vi "Adressen.vi"(8 "error in (no error)":errorcluster caption="Fehler (Eingang, kein Fehler)", 11 "mini8 Steuerung PNS Eingang":refnum<class "mini8 Steuerung PNS.lvclass">) -> (0 "error out":errorcluster caption="Fehler (Ausgang)", 2 "Adressen out":T1, 3 "mini8 Steuerung PNS Ausgang":refnum<class "mini8 Steuerung PNS.lvclass">)   [LabVIEW 2020, in "mini8 Steuerung PNS.lvclass"]
uses:
  mini8 Steuerung PNS.lvclass
  Adresse.ctl
  Steuerung PNS.lvclass
panel:
  out "Alarm":u16[](array[numeric])
  out "Allgemein":u16[](array[numeric])
  out "Heizkreiserkennung":u16[](array[numeric])
  out "Loop1":u16[](array[numeric])
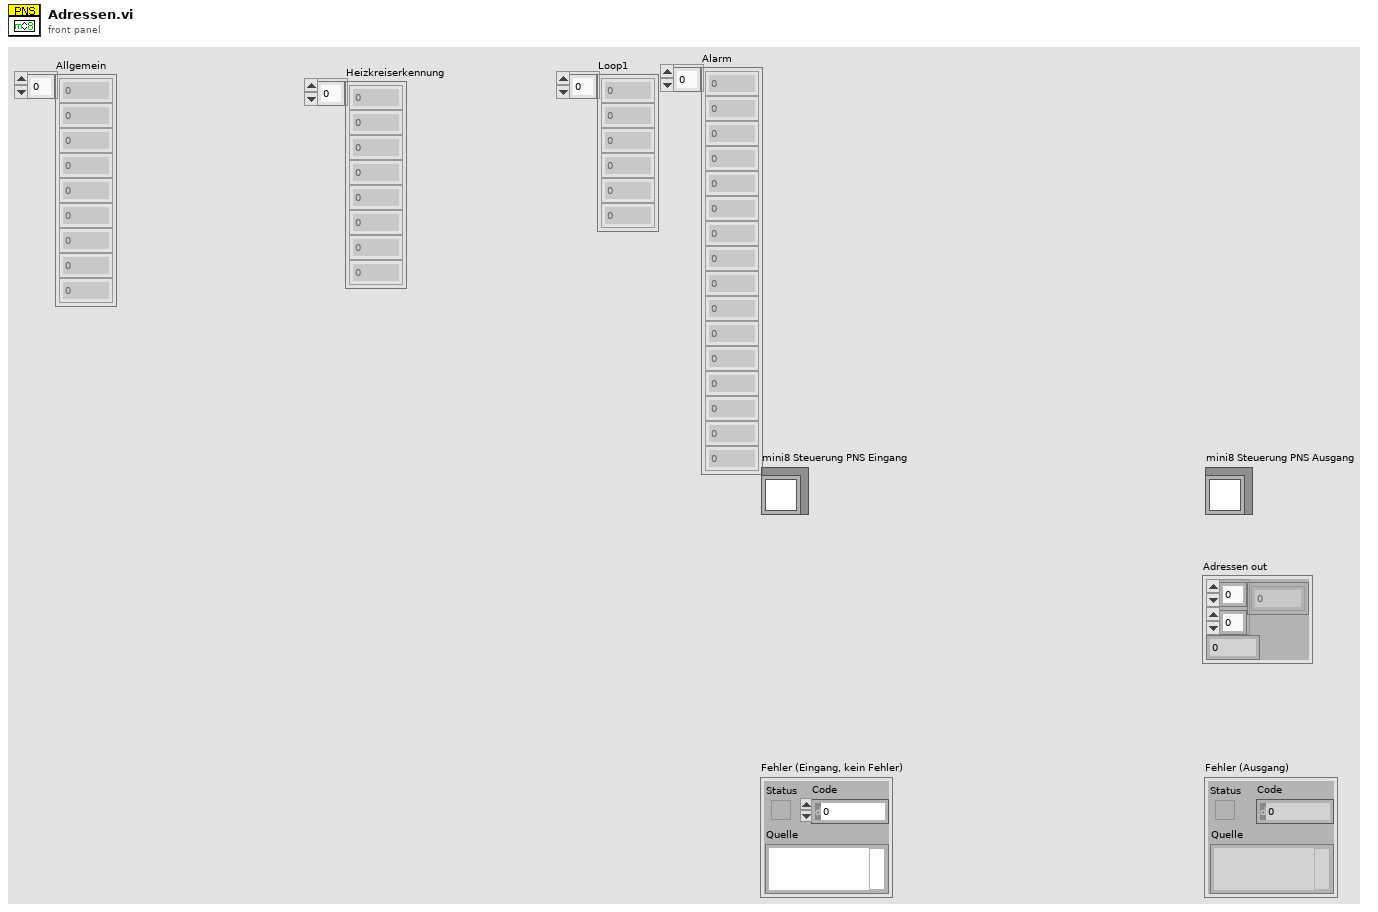
[diagram p1: front panel]
types:
  T1 = typedef "Steuerung PNS.lvclass/Adresse.ctl" = cluster{i32[][], i32}
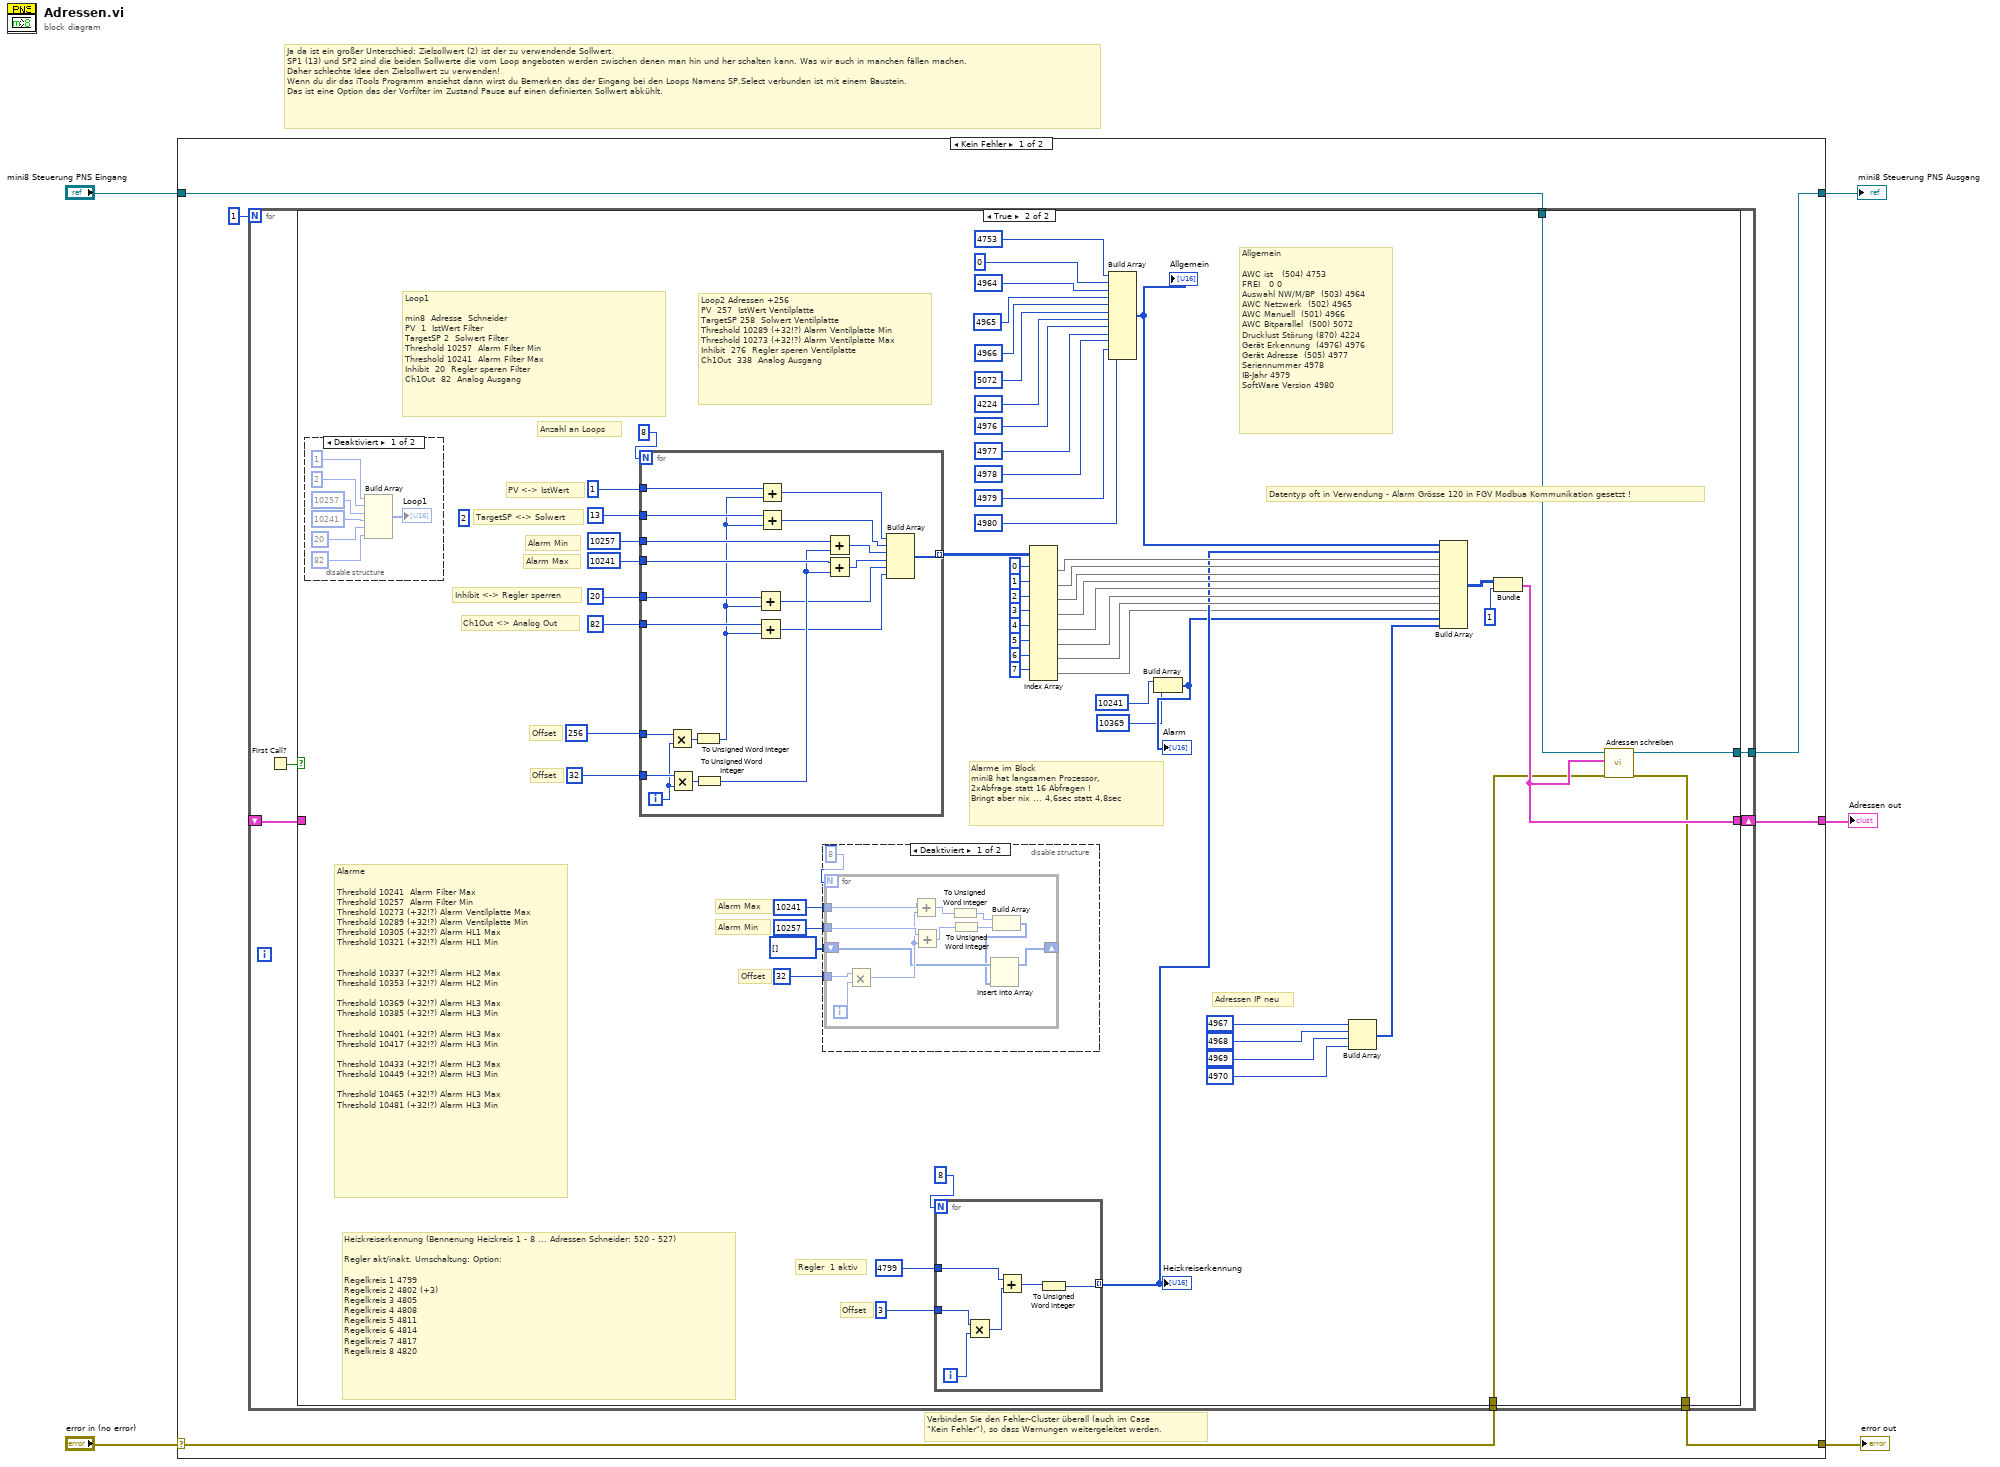
[diagram p0: block diagram]
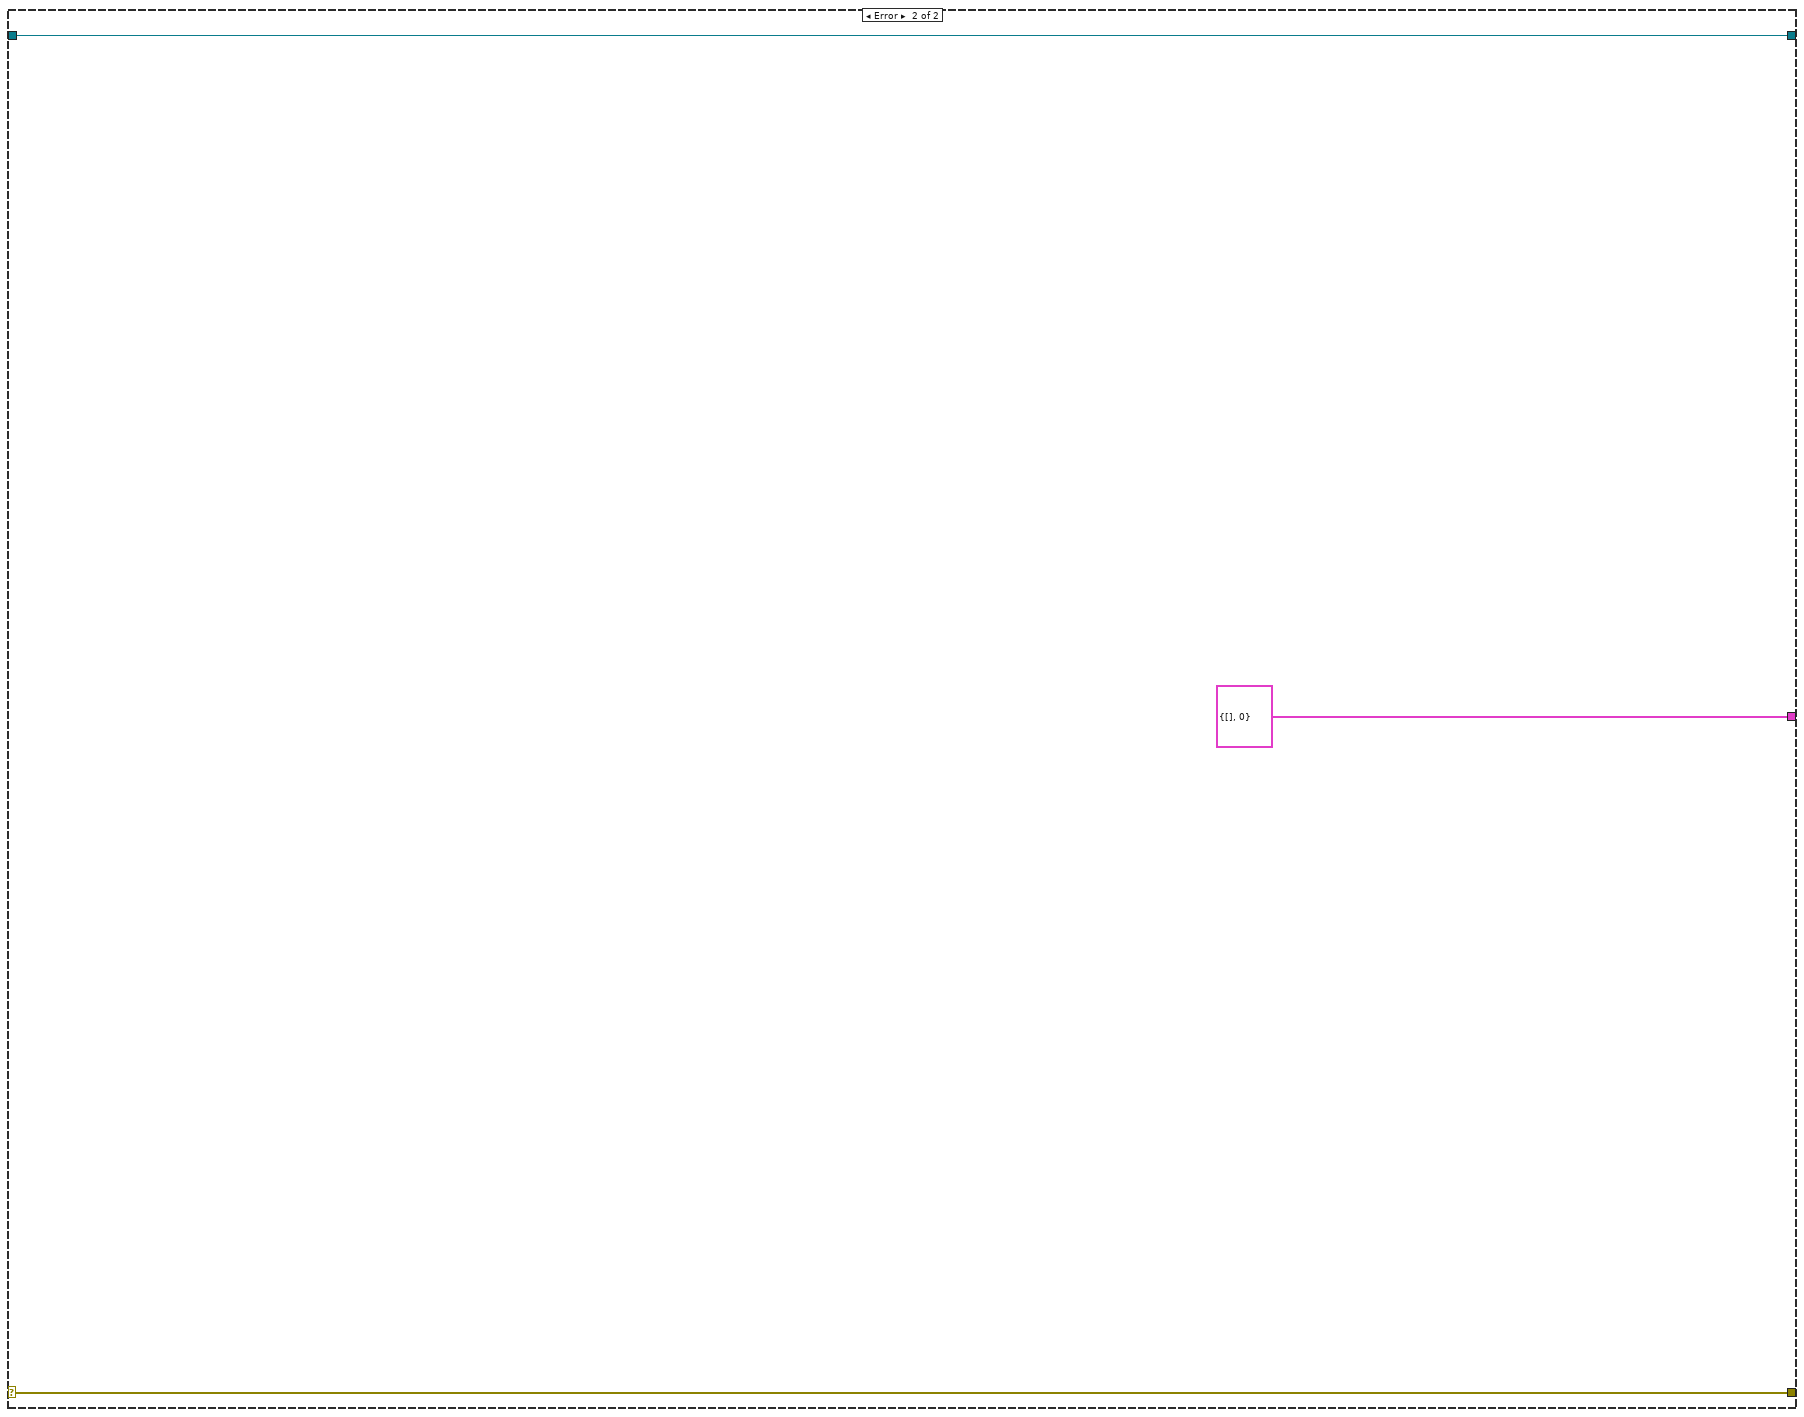
[diagram p5: hidden frame]
diagram:
  # "Ja da ist ein großer Unterschied: Zielsollwert (2) ist der zu verwendende Sollwert.\nSP1 (13) und SP2 sind die beiden Sollwerte die vom Loop angeboten werden zwischen denen man hin und her schalten kann. Was wir auch in manchen fällen machen. \nDaher schlechte Idee den Zielsollwert zu verwenden!\nWenn du dir das iTools Programm ansiehst dann wirst du Bemerken das der Eingang bei den Loops Namens SP.Select verbunden ist mit einem Baustein.\nDas ist eine Option das der Vorfilter im Zustand Pause auf einen definierten Sollwert abkühlt."
  n1 = case shown="Kein Fehler" "error in (no error)" {
    selector: "error in (no error)" -> [w7 w136]
    tunnel: [w6 w136] -> w4
    tunnel: [w8 w135] -> w2
    tunnel: "mini8 Steuerung PNS Eingang" -> [w9 w135]
    tunnel: [w11 cluster{i32[][], i32} {[], 0} ("Adressen out")] -> w1
    frame No Error {
      # "Verbinden Sie den Fehler-Cluster überall (auch im Case\n\"Kein Fehler\"), so dass Warnungen weitergeleitet werden."
      n2 = for {
        N: 1 -> [_]
        shift-right: [w17] -> w11
        shift-left: _ -> [w16]
        tunnel: [w14] -> w8
        tunnel: w9 -> [w15]
        tunnel: w7 -> [w13]
        tunnel: [w12] -> w6
        n3 = First Call?() -> (First Call?: T/F=w18:bool)
        n4 = case shown="True" w18 {
          tunnel: [w21 w35] -> w17
          tunnel: w16 -> [w21 _]
          tunnel: w15 -> [w20 w33]
          tunnel: [w20 w34] -> w14
          tunnel: w13 -> [w19 w32]
          tunnel: [w19 w31] -> w12
          frame False {
          }
          frame True {
            (unwired) u16 2 ("Numerisches Element")
            # "Adressen IP neu"
            # "Datentyp oft in Verwendung - Alarm Grösse 120 in FGV Modbua Kommunikation gesetzt !"
            # "Alarme im Block\nmini8 hat langsamen Prozessor,\n2xAbfrage statt 16 Abfragen !\nBringt aber nix ... 4,6sec statt 4,8sec"
            # "Allgemein\n\nAWC ist\t\t\t(504)\t4753\nFREI\t\t\t0\t0\nAuswahl NW/M/BP\t\t(503)\t4964\nAWC Netzwerk\t\t(502)\t4965\nAWC Manuell\t\t(501)\t4966\nAWC Bitparallel\t\t(500)\t5072\nDrucklust Störung\t(870)\t4224\nGerät Erkennung\t\t(4976)\t4976\nGerät Adresse\t\t(505)\t4977\nSeriennummer 4978\nIB-Jahr 4979\nSoftWare Version 4980"
            # "Offset"
            # "Regler  1 aktiv"
            # "Heizkreiserkennung (Bennenung Heizkreis 1 - 8 ... Adressen Schneider: 520 - 527)\n\nRegler akt/inakt. Umschaltung: Option:\n\nRegelkreis 1\t4799\nRegelkreis 2\t4802 (+3)\nRegelkreis 3\t4805\nRegelkreis 4\t4808\nRegelkreis 5\t4811\nRegelkreis 6\t4814\nRegelkreis 7\t4817\nRegelkreis 8\t4820"
            # "Alarm Min"
            # "Alarm Max"
            # "Offset"
            # "Alarme\n\nThreshold\t10241\t\tAlarm Filter Max\nThreshold\t10257\t\tAlarm Filter Min\nThreshold\t10273\t(+32!?)\tAlarm Ventilplatte Max\nThreshold\t10289\t(+32!?)\tAlarm Ventilplatte Min\nThreshold\t10305\t(+32!?)\tAlarm HL1 Max\nThreshold\t10321\t(+32!?)\tAlarm HL1 Min\n\n\nThreshold\t10337\t(+32!?)\tAlarm HL2 Max\nThreshold\t10353\t(+32!?)\tAlarm HL2 Min\n\nThreshold\t10369\t(+32!?)\tAlarm HL3 Max\nThreshold\t10385\t(+32!?)\tAlarm HL3 Min\n\nThreshold\t10401\t(+32!?)\tAlarm HL3 Max\nThreshold\t10417\t(+32!?)\tAlarm HL3 Min\n\nThreshold\t10433\t(+32!?)\tAlarm HL3 Max\nThreshold\t10449\t(+32!?)\tAlarm HL3 Min\n\nThreshold\t10465\t(+32!?)\tAlarm HL3 Max\nThreshold\t10481\t(+32!?)\tAlarm HL3 Min"
            # "Ch1Out <> Analog Out"
            # "Inhibit <-> Regler sperren"
            # "Alarm Max"
            # "Alarm Min"
            # "TargetSP <-> Solwert"
            # "PV <-> IstWert"
            # "Offset"
            # "Offset"
            # "Loop2 Adressen +256\nPV\t\t257\t\tIstWert Ventilplatte\nTargetSP\t258\t\tSolwert Ventilplatte\nThreshold\t10289\t(+32!?)\tAlarm Ventilplatte Min\nThreshold\t10273\t(+32!?)\tAlarm Ventilplatte Max\nInhibit\t\t276\t\tRegler speren Ventilplatte\nCh1Out\t\t338\t\tAnalog Ausgang"
            # "Anzahl an Loops"
            # "Loop1\n\nmin8\t\tAdresse\t\tSchneider\nPV\t\t1\t\tIstWert Filter\nTargetSP\t2\t\tSolwert Filter\nThreshold\t10257\t\tAlarm Filter Min\nThreshold\t10241\t\tAlarm Filter Max\nInhibit\t\t20\t\tRegler speren Filter\nCh1Out\t\t82\t\tAnalog Ausgang"
            n5 = disable-structure shown="Deaktiviert" {
              frame Disabled {
                n6 = Build Array(u16 1 ("Numerisches Element"), u16 2 ("Numerisches Element"), u16 10257 ("Numerisches Element"), u16 10241 ("Numerisches Element"), u16 20 ("Numerisches Element"), u16 82 ("Numerisches Element")) -> (→"Loop1":u16[])
              }
              frame Enabled {
              }
            }
            n7 = for {
              N: 8 -> [_]
              tunnel: u16 256 ("Numerisches Element") -> [w133]
              tunnel: u16 32 ("Numerisches Element") -> [w131]
              tunnel: u16 1 ("Numerisches Element") -> [w128]
              tunnel: u16 13 ("Numerisches Element") -> [w127]
              tunnel: u16 10257 ("Numerisches Element") -> [w126]
              tunnel: u16 10241 ("Numerisches Element") -> [w125]
              tunnel: u16 20 ("Numerisches Element") -> [w123]
              tunnel: u16 82 ("Numerisches Element") -> [w122]
              tunnel: [w114] -> w74 mode=indexing
              i -> [w130]
              n8 = Multiply(x=w133, y=w130) -> (x*y=w132:i32)
              n9 = Multiply(x=w131, y=w130) -> (x*y=w129:i32)
              n10 = To Unsigned Word Integer(number=w132) -> (unsigned 16bit integer=w121:u16)
              n11 = To Unsigned Word Integer(number=w129) -> (unsigned 16bit integer=w124:u16)
              n12 = Add(x=w123, y=w121) -> (x+y=w116:u16)
              n13 = Add(x=w122, y=w121) -> (x+y=w115:u16)
              n14 = Add(x=w128, y=w121) -> (x+y=w120:u16)
              n15 = Add(x=w127, y=w121) -> (x+y=w119:u16)
              n16 = Add(x=w126, y=w124) -> (x+y=w118:u16)
              n17 = Add(x=w125, y=w124) -> (x+y=w117:u16)
              n18 = Build Array(w120, w119, w118, w117, w116, w115) -> (w114:u16[])
            }
            n19 = disable-structure shown="Deaktiviert" {
              disable-tunnel: u16 32 ("Numerisches Element") -> [w87 _]
              disable-tunnel: u16[] [] -> [w86 _]
              disable-tunnel: u16 10241 ("Numerisches Element") -> [w85 _]
              disable-tunnel: u16 10257 ("Numerisches Element") -> [w84 _]
              frame Disabled {
                n20 = for {
                  N: 8 -> [_]
                  tunnel: w87 -> [w100]
                  tunnel: w85 -> [w98]
                  tunnel: w84 -> [w97]
                  shift-right: [w93] -> _
                  shift-left: w86 -> [w95]
                  i -> [w99]
                  n21 = Multiply(x=w100, y=w99) -> (x*y=w96:i32)
                  n22 = Add(x=w98, y=w96) -> (x+y=w92:i32)
                  n23 = Add(x=w97, y=w96) -> (x+y=w90:i32)
                  n24 = To Unsigned Word Integer(number=w92) -> (unsigned 16bit integer=w91:u16)
                  n25 = To Unsigned Word Integer(number=w90) -> (unsigned 16bit integer=w89:u16)
                  n26 = Build Array(w91, w89) -> (w94:u16[])
                  n27 = Insert Into Array(array=w95, new element=w94) -> (w93:u16[])  [unwired: 1 in]
                }
              }
              frame Enabled {
              }
            }
            n28 = for {
              N: 8 -> [_]
              tunnel: u16 4799 ("Numerisches Element") -> [w104]
              tunnel: u16 3 ("Numerisches Element") -> [w105]
              tunnel: [w101] -> w52 mode=indexing
              i -> [w106]
              n29 = Multiply(x=w105, y=w106) -> (x*y=w103:i32)
              n30 = Add(x=w104, y=w103) -> (x+y=w102:i32)
              n31 = To Unsigned Word Integer(number=w102) -> (unsigned 16bit integer=w101:u16)
            }
            "Heizkreiserkennung" <- w52
            n32 = Index Array(array=w74, index (row) #1=0 ("Index (Zeile)"), index (row) #2=1 ("Index (Zeile)"), index (row) #3=2 ("Index (Zeile)"), index (row) #4=3 ("Index (Zeile)"), index (row) #5=4 ("Index (Zeile)"), index (row) #6=5 ("Index (Zeile)"), index (row) #7=6 ("Index (Zeile)"), index (row) #8=7 ("Index (Zeile)")) -> (element #1=w64:u16[], element #2=w63:u16[], element #3=w62:u16[], element #4=w61:u16[], element #5=w60:u16[], element #6=w59:u16[], element #7=w58:u16[], element #8=w25:u16[])  [unwired: 8 in]
            n33 = Build Array(u16 4753, u16 0, u16 4964, u16 4965, u16 4966, u16 5072, u16 4224, u16 4976, u16 4977, u16 4978, u16 4979, u16 4980) -> (w46:u16[])
            "Allgemein" <- w46
            n34 = Build Array(u16 10241 ("Numerisches Element"), u16 10369 ("Numerisches Element")) -> (w38:u16[])
            "Alarm" <- w38
            n35 = Build Array(u16 4967 ("Numerisches Element"), u16 4968 ("Numerisches Element"), u16 4969 ("Numerisches Element"), u16 4970 ("Numerisches Element")) -> (w26:u16[])
            n36 = Build Array(w46, w52, w64, w63, w62, w61, w60, w59, w58, w25, w38, w26) -> (w73:u16[][])
            n37 = Bundle(w73, u16 1) -> (w35:cluster{u16[][], u16})  [unwired: 1 in]
            n38 = call-dynamic "Adressen schreiben.vi"("error in (no error)"=w32, "Adressen"=w35, "Steuerung PNS (Eingang)"=w33) -> ("error out"=w31:errorcluster, "Steuerung PNS (Ausgang)"=w34:refnum<class "mini8 Steuerung PNS.lvclass">)  [unwired: 7 in]
          }
        }
      }
    }
    frame Error {
    }
  }
  "error out" <- w4
  "mini8 Steuerung PNS Ausgang" <- w2
  "Adressen out" <- w1
